vi "Task5.vi"() -> ()   [LabVIEW 2014, in "Diaz_Excercise_3.lvrbt"]
uses:
  Diaz_Excercise_3.lvrbt
panel:
  out "ERROR?":bool
  out "Current Distance":dbl
  in  "Max Distance":dbl
  in  "Min Distance":dbl
  out "Wall Proximity":string
  out "Distance LED":bool
  in  "stop":bool
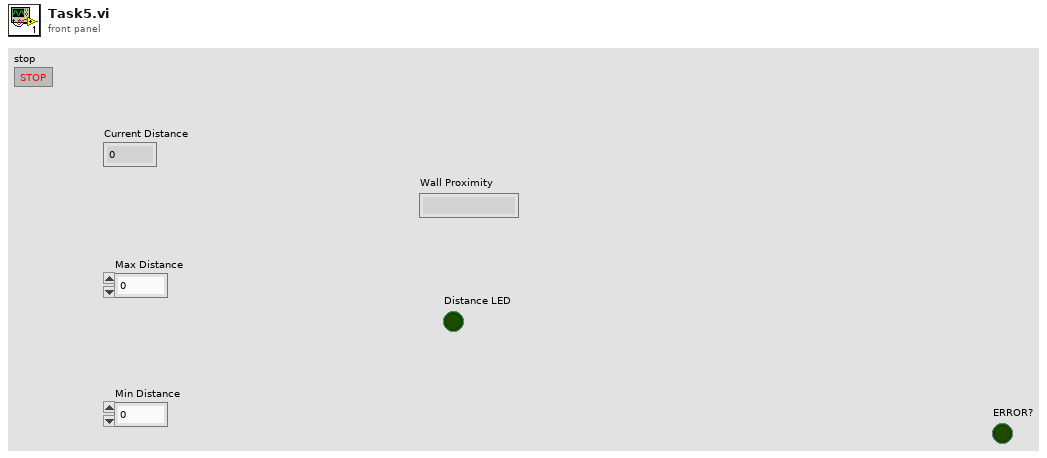
[diagram p1: front panel]
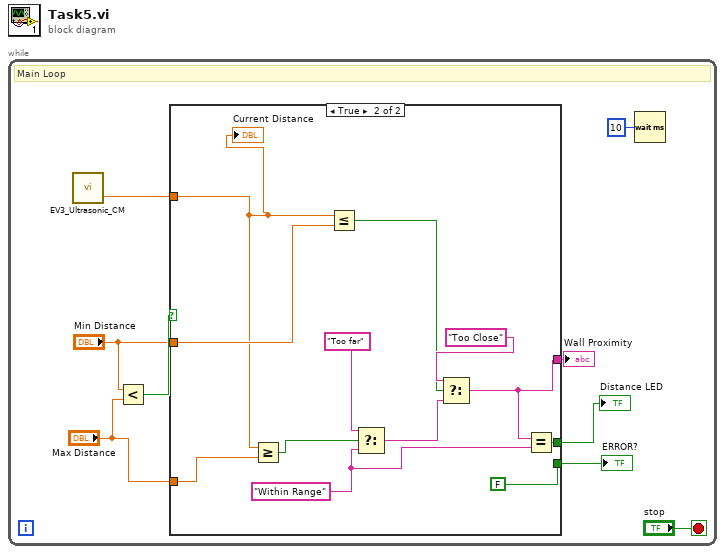
[diagram p0: block diagram]
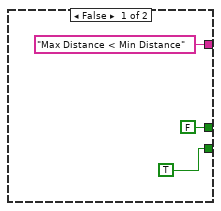
[diagram p2: hidden frame]
diagram:
  n1 = while {
    stop <- "stop" stop-if-true
    # "Main Loop"
    n2 = call <vilib>:"EV3_Ultrasonic_CM.vi"() -> ("Centimeters"=w9:sgl)  [unwired: 3 in, 1 out]
    n3 = Less?(x="Min Distance", y="Max Distance") -> (x < y?=w4:bool)
    n4 = case shown="True" w4 {
      tunnel: "Max Distance" -> [_ w24]
      tunnel: "Min Distance" -> [_ w23]
      tunnel: w9 -> [_ w22]
      tunnel: [FALSE w16] -> w8
      tunnel: ["Max Distance < Min Distance" w15] -> w6
      tunnel: [TRUE FALSE] -> w1
      frame False {
      }
      frame True {
        w19 = "Within Range"
        n5 = Greater Or Equal?(x=w22, y=w24) -> (x >= y?=w21:bool)
        n6 = Less Or Equal?(x=w22, y=w23) -> (x <= y?=w14:bool)
        n7 = Select(t="Too far", s=w21, f=w19) -> (s? t:f=w18:string)
        n8 = Select(t="Too Close", s=w14, f=w18) -> (s? t:f=w15:string)
        n9 = Equal?(x=w15, y=w19) -> (x = y?=w16:bool)
        "Current Distance" <- w22
      }
    }
    "Wall Proximity" <- w6
    "Distance LED" <- w8
    "ERROR?" <- w1
    n10 = Wait (ms)(milliseconds to wait=u32 10) -> ()  [unwired: 1 out]
  }
